vi "DHE_SetBinValues.vi"(8 "error in":errorcluster, 9 "ybin":i32, 10 "xbin":i32) -> (0 "errorout":errorcluster)   [LabVIEW 2016]
uses:
  DBSHAND/private/vis/DatabaseHand_Element_Set(string).vi
  DBSHAND/private/vis/DatabaseHand_Element_Set(I32).vi
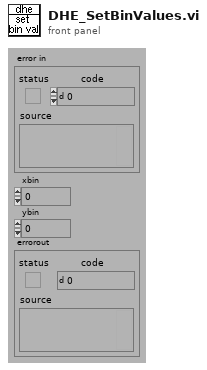
[diagram p1: front panel]
types:
  T1 = typedef "DatabaseHand_RefNum.ctl" = refnum<vi>
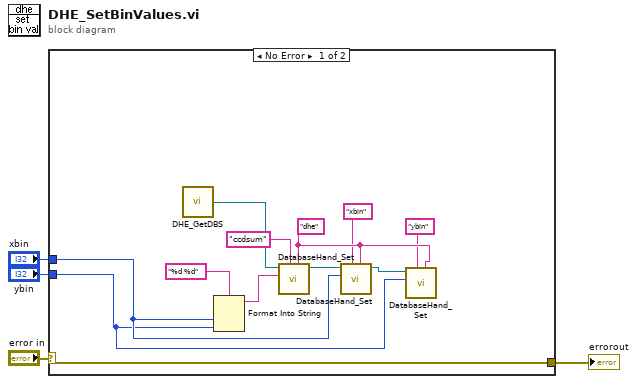
[diagram p0: block diagram]
diagram:
  n1 = case shown="No Error" "error in" {
    selector: "error in" -> [w16 w17]
    tunnel: "xbin" -> [w6 _]
    tunnel: "ybin" -> [w5 _]
    tunnel: [w16 w17] -> w1
    frame No Error {
      w9 = "dhe" ("group")
      n2 = call "DHE_GetDBS.vi"() -> ("DHE_DBSRef"=w12:T1)  [unwired: 9 out]
      n3 = Format Into String(format string="%d %d", w6, w5) -> (resulting string=w13:string)  [unwired: 2 in, 1 out]
      n4 = call-poly "DatabaseHand_Set.vi"("group"=w9, "name"="ccdsum", "value"=w13, "Database RefNum in"=w12) -> ("Database RefNum out"=w11:T1)  [unwired: 4 in, 3 out]
      n5 = call-poly "DatabaseHand_Set.vi"("group"=w9, "name"="xbin", "value"=w6, "Database RefNum in"=w11) -> ("Database RefNum out"=w10:T1)  [unwired: 4 in, 3 out]
      n6 = call-poly "DatabaseHand_Set.vi"("group"=w9, "name"="ybin", "value"=w5, "Database RefNum in"=w10) -> ()  [unwired: 4 in, 4 out]
    }
    frame Error {
    }
  }
  "errorout" <- w1
